vi "background worker.vi"(11 "subscriber in":refnum<class "subscriber.lvclass">) -> ()   [LabVIEW 2015, in "subscriber.lvclass"]
uses:
  subscriber.lvclass
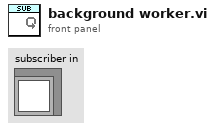
[diagram p1: front panel]
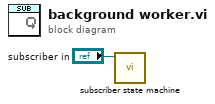
[diagram p0: block diagram]
diagram:
  n1 = call "subscriber state machine.vi"("subscriber"="subscriber in") -> ()  [unwired: 11 in]
